vi "Read Secret.vi"(8 "error in (no error)":errorcluster, 11 "SecretBasedAuthenticatorBase in":refnum<class "SecretBasedAuthenticatorBase.lvclass">) -> (0 "error out":errorcluster, 2 "Secret":string, 3 "SecretBasedAuthenticatorBase out":refnum<class "SecretBasedAuthenticatorBase.lvclass">)   [LabVIEW 2020, in "wamplv.lvlib" / "SecretBasedAuthenticatorBase.lvclass"]
uses:
  SecretBasedAuthenticatorBase.lvclass
  SecretBasedAuthenticatorBase.lvclass/SecretBasedAuthenticatorBase.ctl
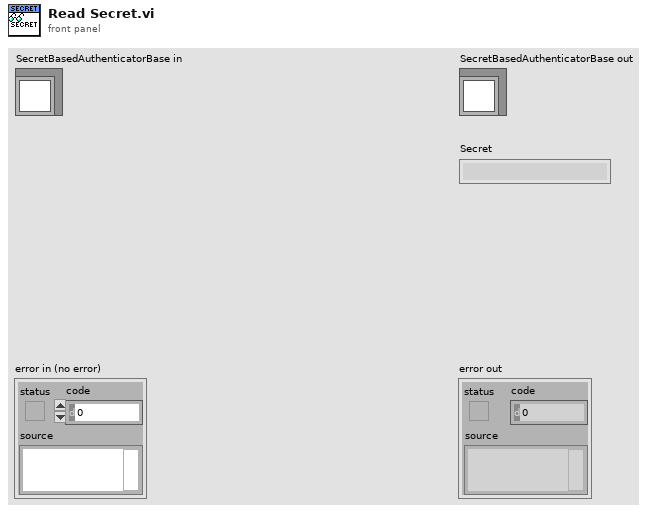
[diagram p1: front panel]
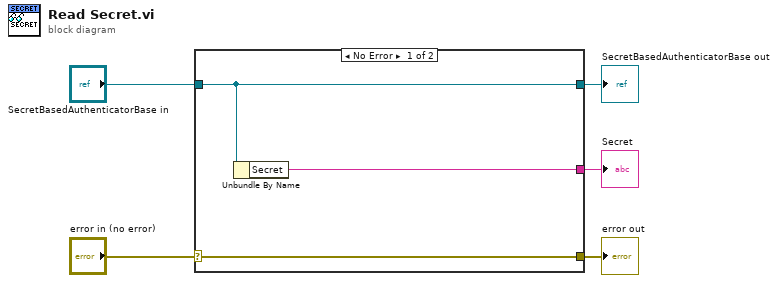
[diagram p0: block diagram]
diagram:
  n1 = case shown="No Error" "error in (no error)" {
    selector: "error in (no error)" -> [w8 w9]
    tunnel: [w8 w9] -> w4
    tunnel: [w7 w10] -> w2
    tunnel: "SecretBasedAuthenticatorBase in" -> [w7 w10]
    tunnel: [w6 _] -> w1
    frame No Error {
      n2 = Unbundle By Name(w7) -> ("Secret"=w6:string)
    }
    frame Error {
    }
  }
  "error out" <- w4
  "SecretBasedAuthenticatorBase out" <- w2
  "Secret" <- w1
